vi "enemies behaviour.vi"(4 "level":i32, 5 "row column orientation every enemy in":cluster{dbl[], dbl[], dbl[]}, 8 "enemies on board":dbl[](array[numeric]), 10 "all enemies in":cluster{u32[][], u32[][], u32[][], u32[][]}={[[0, 11579568, 8553090, 0], [13487565, 8684676, 9539985, 12171705], [9868950, 13290186, 10855845, 11447982], [0, 9211020, 11447982, 0]], [[0, 0, 8355711, 8421504, 0, 0], [0, 13290186, 8816262, 9868950, 11579568, 0], [13290186, 9868950, 7631988, 8684676, 11316396, 8487297], [8947848, 11121611, 5987163, 11447982, 12369084, 7171459], [0, 9868950, 7105644, 9868950, 9868950, 0], [0, 0, 9868950, 5855577, 0, 0]], [[0, 0, 0, 0, 9013641, 11974326, 0, 0, 0, 0], [0, 0, 12434877, 10395294, 12434877, 4079166, 12369084, 11184810, 0, 0], [0, 10921638, 10395294, 8355711, 10395294, 10000536, 13750737, 11908533, 11053224, 0], [0, 11711154, 12961221, 13487565, 11711154, 9145227, 12500670, 12040119, 7763574, 0], [11711154, 13750737, 12698049, 12763842, 9605778, 7763574, 4276545, 10263708, 13027014, 10461087], [14606046, 12632256, 12895428, 11842740, 9013641, 7631988, 6316128, 7039851, 12369084, 10987431], [0, 11053224, 13619151, 10855845, 6118749, 8092539, 8816262, 8421504, 11579568, 0], [0, 11119017, 10921638, 12698049, 8355711, 9474192, 10987431, 11579568, 11579568, 0], [0, 0, 12040119, 11776947, 10000536, 11908533, 9605778, 10132122, 0, 0], [0, 0, 0, 0, 12171705, 12500670, 0, 0, 0, 0]], [[0, 0, 1190399, 0, 0], [0, 1190399, 2472704, 1190399, 0], [13290186, 12369084, 11316396, 12369084, 11316396], [0, 11121611, 11776947, 11121611, 0], [0, 0, 0, 0, 0]]}, 11 "Board with missles in":u32[][](array[numeric])) -> (0 "enemies on board out":dbl[](array[numeric]), 1 "row column orientation every enemy out":cluster{dbl[], dbl[], dbl[]}, 2 "level out":i32, 3 "Board with enemies":u32[][](array[numeric]))   [LabVIEW 2019]
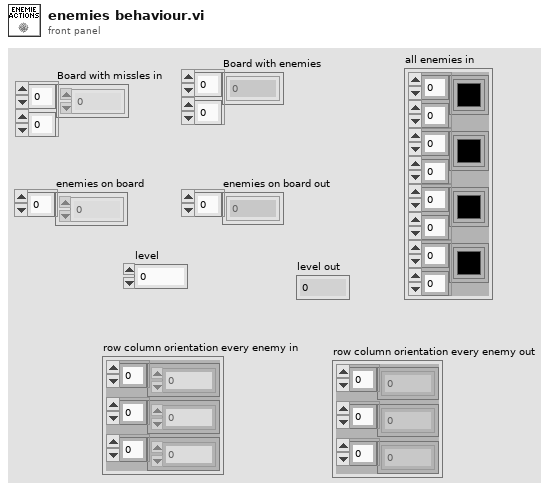
[diagram p1: front panel]
types:
  T1 = cluster{"new row":dbl[], "new column":dbl[], "orientation":dbl[]}
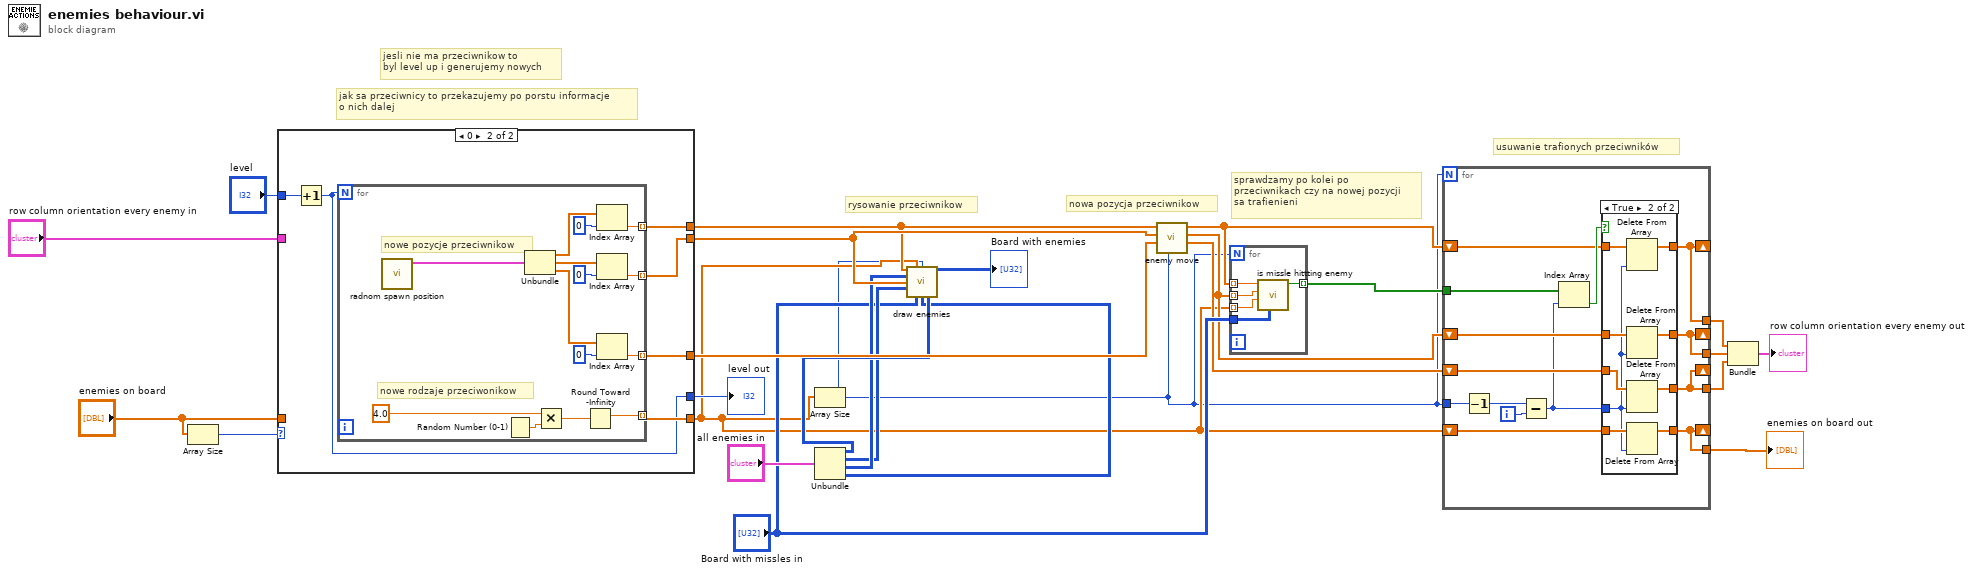
[diagram p0: block diagram]
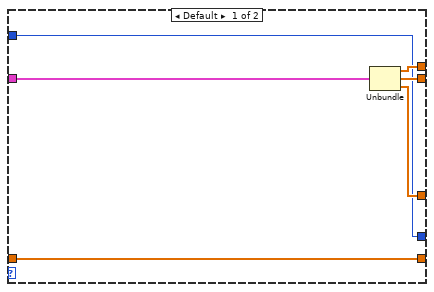
[diagram p3: hidden frame]
diagram:
  # "usuwanie trafionych przeciwników"
  # "nowa pozycja przeciwnikow"
  # "rysowanie przeciwnikow"
  # "jesli nie ma przeciwnikow to\nbyl level up i generujemy nowych"
  # "jak sa przeciwnicy to przekazujemy po porstu informacje\no nich dalej"
  # "sprawdzamy po kolei po\nprzeciwnikach czy na nowej pozycji\nsa trafienieni"
  n1 = Array Size(array="enemies on board") -> (size(s)=w11:i32)
  n2 = case shown="0" w11 {
    tunnel: [w32 w38] -> w2
    tunnel: "enemies on board" -> [w32 _]
    tunnel: "level" -> [w27 w34]
    tunnel: [w30 w37] -> w19
    tunnel: [w29 w36] -> w20
    tunnel: "row column orientation every enemy in" -> [w31 _]
    tunnel: [w28 w35] -> w21
    tunnel: [w27 w33] -> w3
    frame Default {
      n3 = Unbundle(w31) -> (w30:dbl[], w29:dbl[], w28:dbl[])
    }
    frame 0 {
      n4 = Increment(x=w34) -> (x+1=w33:i32)
      n5 = for {
        N: w33 -> [_]
        tunnel: [w49] -> w38 mode=indexing
        tunnel: [w39] -> w37 mode=indexing
        tunnel: [w40] -> w36 mode=indexing
        tunnel: [w41] -> w35 mode=indexing
        # "nowe pozycje przeciwnikow"
        # "nowe rodzaje przeciwonikow"
        n6 = call "radnom spawn position.vi"() -> ("cluster of arrays of enemie data"=w48:cluster{dbl[], dbl[], dbl[]})  [unwired: 11 in]
        n7 = Random Number (0-1)() -> (number: 0 to 1=w51:dbl)
        n8 = Unbundle(w48) -> (w47:dbl[], w46:dbl[], w45:dbl[])
        n9 = Multiply(x=4.0, y=w51) -> (x*y=w52:dbl)
        n10 = Round Toward -Infinity(1:w52) -> (0:w49:dbl)
        n11 = Index Array(array=w47, index=0) -> (element=w39:dbl)
        n12 = Index Array(array=w46, index=0) -> (element=w40:dbl)
        n13 = Index Array(array=w45, index=0) -> (element=w41:dbl)
      }
    }
  }
  "level out" <- w3
  n14 = Array Size(array=w2) -> (size(s)=w1:i32)
  n15 = Unbundle("all enemies in") -> (w17:u32[][], w15:u32[][], w16:u32[][], w14:u32[][])
  n16 = call "draw enemies.vi"("Array of rows for every enemy"=w19, "enemies on board"=w2, "number of enemies"=w1, "big rock"=w16, "array of columns for every enemy"=w20, "rock"=w15, "blank Board in"="Board with missles in", "UFO Ship"=w14, "small rock"=w17) -> ("Board with enemies out"=→"Board with enemies":u32[][])  [unwired: 6 in]
  n17 = call "enemy move.vi"("number of enemies"=w1, "orientation"=w21, "column"=w20, "row"=w19) -> ("orientation"=w8:dbl[], "new column"=w9:dbl[], "new row"=w10:dbl[])  [unwired: 5 in]
  n18 = for {
    N: w1 -> [_]
    tunnel: "Board with missles in" -> [w54]
    tunnel: w9 -> [w56] mode=indexing
    tunnel: w10 -> [w55] mode=indexing
    tunnel: w2 -> [w57] mode=indexing
    tunnel: [w53] -> w12 mode=indexing
    n19 = call "is missle hittting enemy.vi"("Board with missles in"=w54, "enemy type"=w57, "colum"=w56, "row"=w55) -> ("Boolean"=w53:bool)  [unwired: 7 in]
  }
  n20 = for {
    N: w1 -> [_]
    tunnel: w12 -> [w68]
    tunnel: w1 -> [w69]
    shift-right: [w61] -> _
    shift-left: w10 -> [w66]
    shift-right: [w60] -> _
    shift-left: w9 -> [w65]
    shift-right: [w59] -> _
    shift-left: w8 -> [w64]
    shift-right: [w58] -> _
    shift-left: w2 -> [w63]
    tunnel: [w61] -> w6
    tunnel: [w60] -> w5
    tunnel: [w59] -> w4
    tunnel: [w58] -> w7
    i -> [w71]
    n21 = Decrement(x=w69) -> (x-1=w70:i32)
    n22 = Subtract(x=w70, y=w71) -> (x-y=w62:i32)
    n23 = Index Array(array=w68, index=w62) -> (element=w67:bool)
    n24 = case shown="True" w67 {
      tunnel: w66 -> [w75 w84]
      tunnel: w65 -> [w74 w83]
      tunnel: w64 -> [w73 w82]
      tunnel: w63 -> [w72 w81]
      tunnel: [w75 w79] -> w61
      tunnel: [w74 w78] -> w60
      tunnel: [w73 w77] -> w59
      tunnel: [w72 w76] -> w58
      tunnel: w62 -> [_ w80]
      frame False {
      }
      frame True {
        n25 = Delete From Array(array=w84, index=w80) -> (array with subset deleted=w79:dbl[])  [unwired: 1 in, 1 out]
        n26 = Delete From Array(array=w83, index=w80) -> (array with subset deleted=w78:dbl[])  [unwired: 1 in, 1 out]
        n27 = Delete From Array(array=w82, index=w80) -> (array with subset deleted=w77:dbl[])  [unwired: 1 in, 1 out]
        n28 = Delete From Array(array=w81, index=w80) -> (array with subset deleted=w76:dbl[])  [unwired: 1 in, 1 out]
      }
    }
  }
  "enemies on board out" <- w7
  n29 = Bundle("new row"=w6, "new column"=w5, "orientation"=w4) -> (→"row column orientation every enemy out":T1)  [unwired: 1 in]
